vi "RSZVB Configure Frequency Settings.vi"(5 "Fixed Frequency Signal (0: RF)":i32(ring) items=["RF"=0, "IF"=2, "LO 1"=3, "LO 2"=4], 6 "Frequency Conversion Mode (1: IF = RF – LO)":i32(ring) items=["IF = LO – RF", "IF = RF – LO", "IF = LO + RF"], 7 "Fixed Frequency (300000.0 Hz)":dbl=300000.0 format="%^.3e", 8 "error in (no error)":errorcluster {"code" format="%.0x"}, 9 "Fundamental Frequency Signal (0: RF)":i32(ring) items=["RF"=0, "IF"=2, "LO 1"=3, "LO 2"=4], 10 "Channel (1)":i32=1, 11 "VISA session":refnum<visa-resource-name>) -> (0 "error out":errorcluster {"code" format="%.0x"}, 3 "dup VISA session":refnum<visa-resource-name>)   [LabVIEW 2011]
doc: "This VI configures the frequency settings for the mixer measurement.\n\nRemote-control command(s):\n[SENSe<Ch>:]FREQuency:CONVersion:MIXer:FUNDamental RF | LO | IF\n[SENSe<Ch>:]FREQuency:CONVersion:MIXer:FIXed RF | LO | IF\n[SENSe<Ch>:]FREQuency:CONVersion:MIXer:FFIXed <fixed_frequency>\n[SENSe<Ch>:]FREQuency:CONVersion:MIXer:TFRequency DCLower | DCUPper | UCONversion"
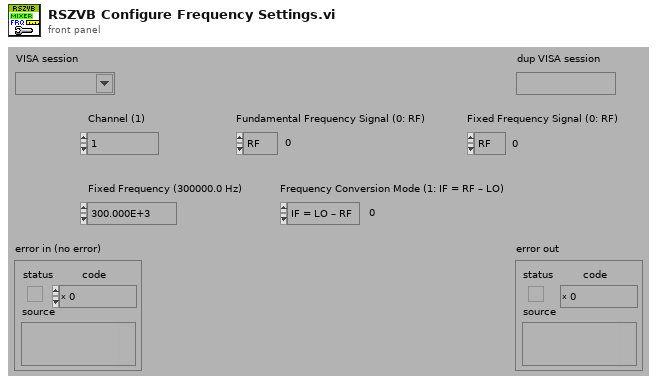
[diagram p1: front panel]
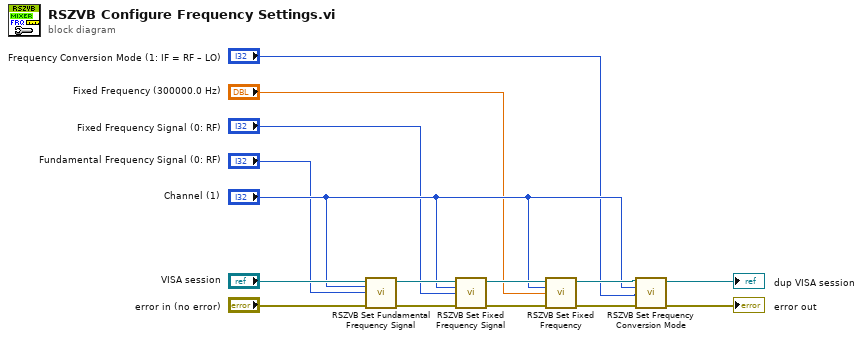
[diagram p0: block diagram]
diagram:
  n1 = call "RSZVB Set Fundamental Frequency Signal.vi"("error in (no error)"="error in (no error)", "Fundamental Frequency (0: RF)"="Fundamental Frequency Signal (0: RF)", "Channel (1)"="Channel (1)", "VISA session"="VISA session") -> ("error out"=w12:errorcluster, "dup VISA session"=w13:refnum<visa-resource-name>)  [unwired: 6 in]
  n2 = call "RSZVB Set Fixed Frequency Signal.vi"("error in (no error)"=w12, "Fixed Frequency (0: RF)"="Fixed Frequency Signal (0: RF)", "Channel (1)"="Channel (1)", "VISA session"=w13) -> ("error out"=w10:errorcluster, "dup VISA session"=w11:refnum<visa-resource-name>)  [unwired: 6 in]
  n3 = call "RSZVB Set Fixed Frequency.vi"("error in (no error)"=w10, "Fixed Frequency (300000.0 Hz)"="Fixed Frequency (300000.0 Hz)", "Channel (1)"="Channel (1)", "VISA session"=w11) -> ("error out"=w8:errorcluster, "dup VISA session"=w9:refnum<visa-resource-name>)  [unwired: 6 in]
  n4 = call "RSZVB Set Frequency Conversion Mode.vi"("error in (no error)"=w8, "Frequency Conversion Mode (1: IF = RF – LO)"="Frequency Conversion Mode (1: IF = RF – LO)", "Channel (1)"="Channel (1)", "VISA session"=w9) -> ("error out"=→"error out":errorcluster, "dup VISA session"=→"dup VISA session":refnum<visa-resource-name>)  [unwired: 6 in]
